vi "Program load indicators.vi"() -> ()   [LabVIEW 2016]
panel:
  out "Coincidence hunt limit":i32
  out "Reads per TDC call":i32
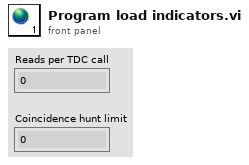
[diagram p1: front panel]
diagram:
